vi "SetMOTFEncoderRate.vi"(8 "error in (no error)":errorcluster, 10 "MOTF encoder rate":i16 caption="MOTF encoder rate [bits/encoderCount]", 11 "SM1000-control in":T1) -> (0 "error out":errorcluster, 3 "SM1000-control out":T1)   [LabVIEW 2013, in "EC1000-control.lvlib" / "SM1000-control.lvclass"]
doc: "Sets the calibration factor used to convert encoder counts to laser galvo command bits (bits/encoderCount).\n\nThe encoder rate relates encoder counts to how far an object travels in the lens field in galvo command bits.\n\nCommand: <\"SetMOTFEncoderRate\">,<rate> or 21,<rate>\nReturns: \"0\""
uses:
  SM1000-control.lvclass
  Object-reference.ctl
  SM1000-control.lvclass/SM1000-control.ctl
  Custom-errors.ctl
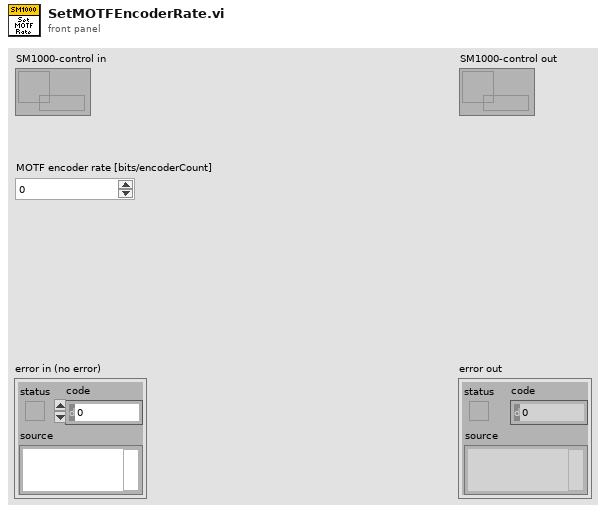
[diagram p1: front panel]
types:
  T1 = typedef "EC1000-control.lvlib/SM1000-control.lvclass/Object-reference.ctl" = refnum<data-value>
  T2 = typedef "EC1000-control.lvlib/SM1000-control.lvclass/Custom-errors.ctl" = enum16{"No error", "Not implemented", "Command not recognized", "Invalid input", "No connection", "Timeout", "Resource not loaded"}
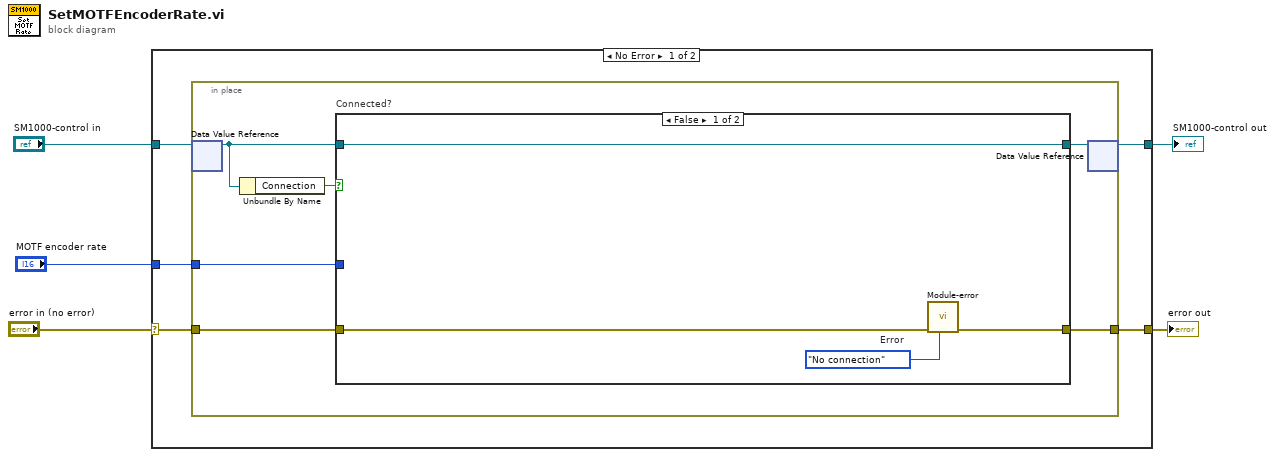
[diagram p0: block diagram]
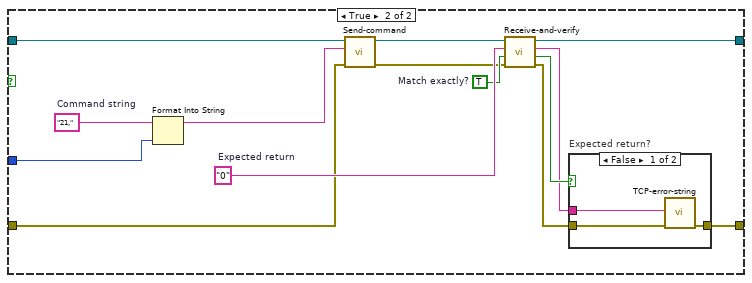
[diagram p2: hidden frame]
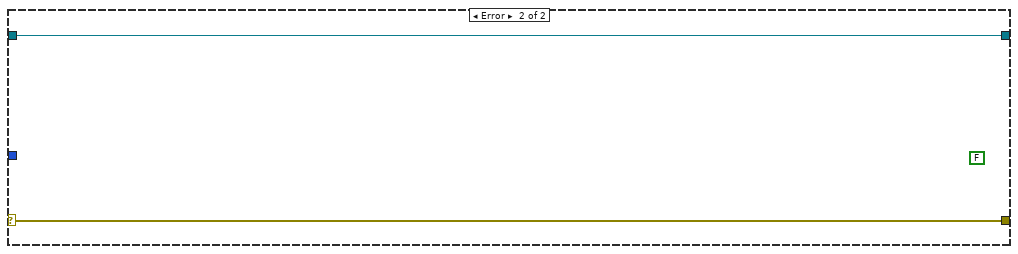
[diagram p4: hidden frame]
diagram:
  n1 = case shown="No Error" "error in (no error)" {
    selector: "error in (no error)" -> [w8 w40]
    tunnel: [w7 w40] -> w4
    tunnel: [w9 w39] -> w2
    tunnel: "SM1000-control in" -> [w10 w39]
    tunnel: "MOTF encoder rate" -> [w6 _]
    frame No Error {
      n2 = in-place {
        in-place-border: w8 -> [w16]
        in-place-border: [w13] -> w7
        in-place-border: w6 -> [w11]
        n3 = in-place-dvr #1(w10) -> (w14:refnum<class "SM1000-control.lvclass">)  [unwired: 1 out]
        n4 = Unbundle By Name(w14) -> ("Connection"=w15:bool)
        n5 = case "Connected?" shown="False" w15 {
          tunnel: w16 -> [w20 w27]
          tunnel: w14 -> [w18 w34]
          tunnel: [w19 w25] -> w13
          tunnel: [w18 w24] -> w12
          tunnel: w11 -> [_ w21]
          frame False {
            w17 = Custom-errors."No connection"  # Error
            n6 = call "Module-error.vi"("Error"=w17, "error in (no error)"=w20) -> ("error out"=w19:errorcluster)  [unwired: 9 in]
          }
          frame True {
            w31 = TRUE  # Match exactly?
            w32 = "0"  # Expected return
            w23 = "21,"  # Command string
            n7 = Format Into String(initial string=w23, w21) -> (resulting string=w22:string)  [unwired: 2 in, 1 out]
            n8 = call "Send-command.vi"("error in (no error)"=w27, "Command string"=w22, "SM1000-control in"=w34) -> ("error out"=w30:errorcluster, "SM1000-control out"=w33:refnum<class "SM1000-control.lvclass">)  [unwired: 7 in]
            n9 = call "Receive-and-verify.vi"("error in (no error)"=w30, "Match exactly?"=w31, "Expected return string"=w32, "SM1000-control in"=w33) -> ("error out"=w26:errorcluster, "Verified?"=w29:bool, "Return string"=w28:string, "SM1000-control out"=w24:refnum<class "SM1000-control.lvclass">)  [unwired: 4 in]
            n10 = case "Expected return?" shown="False" w29 {
              tunnel: w28 -> [w37 _]
              tunnel: w26 -> [w36 w38]
              tunnel: [w35 w38] -> w25
              frame False {
                n11 = call "TCP-error-string.vi"("error in (no error)"=w36, "Retun code"=w37) -> ("error out"=w35:errorcluster)  [unwired: 9 in]
              }
              frame True {
              }
            }
          }
        }
        n12 = in-place-dvr #1(w12) -> (w9:T1)  [unwired: 1 out]
      }
    }
    frame Error {
      (unwired) FALSE
    }
  }
  "error out" <- w4
  "SM1000-control out" <- w2
